vi "MissionSetpoints.vi"() -> (2 "Setpoints Out":T1)   [LabVIEW 2011]
uses:
  2 Typedefs/setpoints to arbiter.ctl
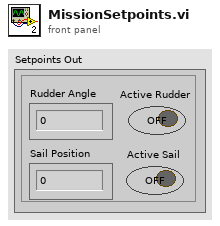
[diagram p1: front panel]
types:
  T1 = typedef "setpoints to arbiter.ctl" = cluster{"Rudder Angle":dbl, "Sail Position":dbl, "Active Rudder":bool, "Active Sail":bool}
  T2 = typedef "sail setpt.ctl" = dbl
  T3 = typedef "heading.ctl" = dbl
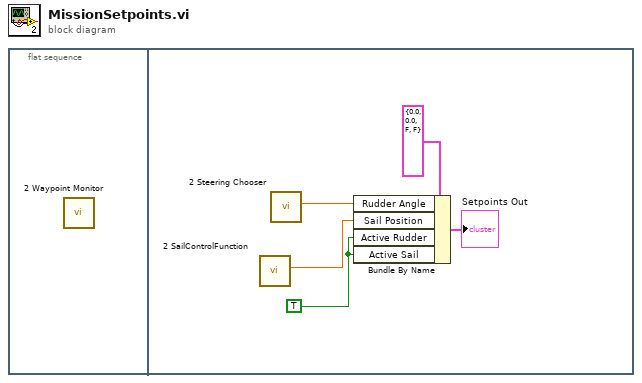
[diagram p0: block diagram]
diagram:
  n1 = flat-sequence {
    frame #0 {
      n2 = call "2 Waypoint Monitor.vi"() -> ()  [unwired: 12 in]
    }
    frame #1 {
      w1 = TRUE
      n3 = call "2 SailControlFunction.vi"() -> ("Sail Position"=w3:T2)  [unwired: 11 in]
      n4 = call "2 Steering Chooser.vi"() -> ("Rudder Angle"=w2:T3)  [unwired: 11 in]
      n5 = Bundle By Name(cluster=T1 {"Rudder Angle"=0.0, "Sail Position"=0.0, "Active Rudder"=FALSE, "Active Sail"=FALSE} ("Setpoints Out"), "Rudder Angle"=w2, "Sail Position"=w3, "Active Rudder"=w1, "Active Sail"=w1) -> (→"Setpoints Out":T1)
    }
  }
